vi "Swap array adjacent elements(I16).vi"(7 "Swap?":bool=TRUE, 10 "Index":i32, 11 "Input":i16[](array[numeric])) -> (3 "Output":i16[](array[numeric]))   [LabVIEW 2012]
doc: "功能：\n\n交换数组相邻两个元素的值，常见于数组冒泡排序中。\n\nSwap?1布尔输入端子用来选择交换数组的相邻元素，默认为FALSE，不交换。\n\nX[i+1]-->X[i]\n\nX[i]---->X[i+1]\n\ncsxcs_366创建"
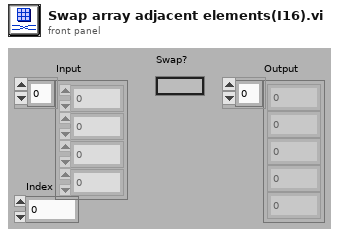
[diagram p1: front panel]
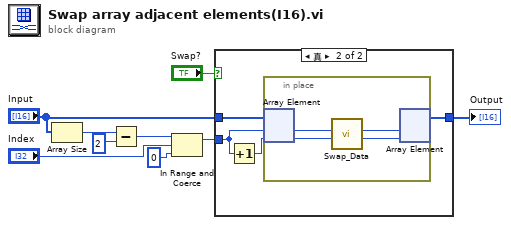
[diagram p0: block diagram]
diagram:
  n1 = Array Size(array="Input") -> (size(s)=w9:i32)
  n2 = Subtract(x=w9, y=2) -> (x-y=w7:i32)
  n3 = In Range and Coerce(upper limit=w7, x="Index", lower limit=0 ("下限")) -> (coerced(x)=w2:i32)  [unwired: 1 out]
  n4 = case shown="真" "Swap?" {
    tunnel: "Input" -> [w10 w14]
    tunnel: w2 -> [_ w12]
    tunnel: [w10 w13] -> w1
    frame False {
    }
    frame True {
      n5 = Increment(x=w12) -> (x+1=w11:i32)
      n6 = in-place {
        n7 = in-place-array #1(w14, w12, w11) -> (w18:i16, w17:i16)
        n8 = call-poly "Swap_Data.vi"("b"=w17, "a"=w18) -> ("b"=w15:i16, "a"=w16:i16)  [unwired: 5 in]
        n9 = in-place-array #1(w16, w15) -> (w13:i16[])  [unwired: 2 out]
      }
    }
  }
  "Output" <- w1
